vi "Read Measurement(Multiple Points).vi"(0 "VISA resource name":refnum<visa-resource-name>, 5 "Trigger Count (1)":dbl=1.0, 7 "Maximum Time (10000 ms)":u32=10000, 11 "error in (no error)":errorcluster) -> (4 "VISA resource name out":refnum<visa-resource-name>, 6 "Measurements":sgl[](array[numeric]), 15 "error out":errorcluster)   [LabVIEW 2020, in "3458A Basic Driver.lvlib"]
doc: "Reads and returns multiple measurements from the instrument. Note that setting the trigger count will cause the multimeter to start taking measurements(except in cases of using an external or level trigger in which case it waits for the adequate input signal). Set an adequate amount in the Maximum Time control to give the DMM enough time to acquire all measurements. The greater the amount of measurements, then the greater the maximum time will be."
uses:
  3458A Basic Driver.lvlib
  Low Level/Fetch Measurement(Multiple Points).vi
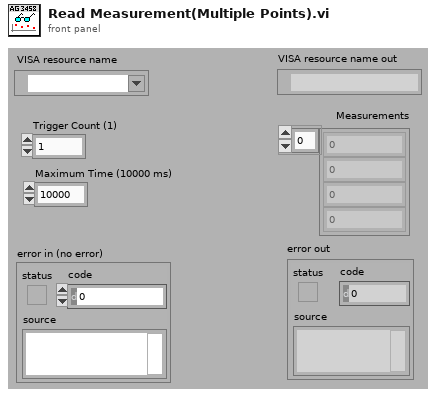
[diagram p1: front panel]
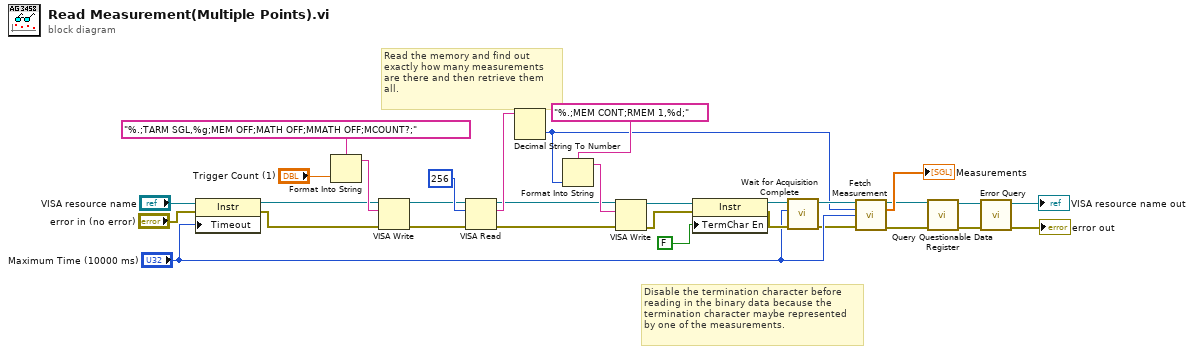
[diagram p0: block diagram]
diagram:
  # "Disable the termination character before\nreading in the binary data because the \ntermination character maybe represented\nby one of the measurements."
  # "Read the memory and find out\nexactly how many measurements\nare there and then retrieve them\nall."
  n1 = property on="Property Node" class="Instr"(reference="VISA resource name", error in="error in (no error)", "Timeout"="Maximum Time (10000 ms)") -> (reference out=w13:refnum<visa-resource-name>, error out=w12:errorcluster)
  n2 = Format Into String(format string="%.;TARM SGL,%g;MEM OFF;MATH OFF;MMATH OFF;MCOUNT?;", "Trigger Count (1)") -> (resulting string=w28:string)  [unwired: 2 in, 1 out]
  n3 = VISA Write(VISA resource name=w13, write buffer=w28, error in (no error)=w12) -> (VISA resource name out=w6:refnum<visa-resource-name>, error out=w5:errorcluster)  [unwired: 1 out]
  n4 = VISA Read(VISA resource name=w6, byte count=u32 256, error in (no error)=w5) -> (VISA resource name out=w23:refnum<visa-resource-name>, read buffer=w26:string, error out=w22:errorcluster)  [unwired: 1 out]
  n5 = Decimal String To Number(string=w26) -> (number=w14:i32)  [unwired: 2 in, 1 out]
  n6 = Format Into String(format string="%.;MEM CONT;RMEM 1,%d;", w14) -> (resulting string=w24:string)  [unwired: 2 in, 1 out]
  n7 = VISA Write(VISA resource name=w23, write buffer=w24, error in (no error)=w22) -> (VISA resource name out=w21:refnum<visa-resource-name>, error out=w20:errorcluster)  [unwired: 1 out]
  n8 = property on="Property Node" class="Instr"(reference=w21, error in=w20, "TermChar En"=FALSE) -> (reference out=w19:refnum<visa-resource-name>, error out=w18:errorcluster)
  n9 = call "Wait for Acquisition Complete.vi"("error in (no error)"=w18, "Maximum Time (10000 ms)"="Maximum Time (10000 ms)", "VISA resource name"=w19) -> ("error out"=w2:errorcluster, "VISA resource name out"=w15:refnum<visa-resource-name>)  [unwired: 7 in]
  n10 = call-poly "Fetch Measurement.vi"("VISA resource name"=w15, "Number Of Readings (1)"=w14, "Timeout Value(10000 ms)"="Maximum Time (10000 ms)", "error in (no error)"=w2) -> ("VISA resource name out"=w9:refnum<visa-resource-name>, "Measurements"=→"Measurements":sgl[], "error out"=w1:errorcluster)  [unwired: 9 in]
  n11 = call "Query Questionable Data Register.vi"("error in (no error)"=w1, "VISA resource name"=w9) -> ("error out"=w7:errorcluster, "VISA resource name out"=w8:refnum<visa-resource-name>)  [unwired: 7 in, 1 out]
  n12 = call "Error Query.vi"("error in (no error)"=w7, "VISA resource name"=w8) -> ("error out"=→"error out":errorcluster, "VISA resource name out"=→"VISA resource name out":refnum<visa-resource-name>)  [unwired: 6 in, 2 out]
